vi "add_channel.vi"(8 "error in (no error)":errorcluster, 11 "Channel definition in":T1={"physical Channel"="", "max_input_value"=0.0, "min_input_value"=0.0, "ground_reference"=10083, "translation_factor"=0.0, "translation_offset"=0.0} {"ground_reference" items=["default"=-1, "RSE"=10083, "NRSE"=10078, "Differential"=10106, "Pseudodifferential"=12529]}) -> (0 "error out":errorcluster, 2 "Canceled":bool, 3 "Channel definition out":T1={"physical Channel"="", "max_input_value"=0.0, "min_input_value"=0.0, "ground_reference"=10083, "translation_factor"=0.0, "translation_offset"=0.0} {"ground_reference" items=["default"=-1, "RSE"=10083, "NRSE"=10078, "Differential"=10106, "Pseudodifferential"=12529]})   [LabVIEW 2012, in "SignalReaderCN091129DAQmx.lvclass"]
doc: "Collects the information to add/edit an Analog input DAQ channel"
uses:
  SignalReaderCN091129DAQmx.lvclass
  C:/Program Files (x86)/National Instruments/LabVIEW 2010/resource/objmgr/daqmx.rc
  TypeDefs/channel_definition_cluster.ctl
panel:
  in  "ground reference":i32(ring)=10083 items=["default"=-1, "RSE"=10083, "NRSE"=10078, "Differential"=10106, "Pseudodifferential"=12529]
  in  "Add":bool
  in  "cancel":bool
  in  "voltage range":i32(ring) items=["-0.20 - 0.20", "-1.00 - 1.00", "-5.00 - 5.00", "-10.00 - 10.00"]
  in  "translation offset":dbl
  in  "translation factor":dbl
  in  "Physical Channel":tag
  # "Add / Edit analog input channel"
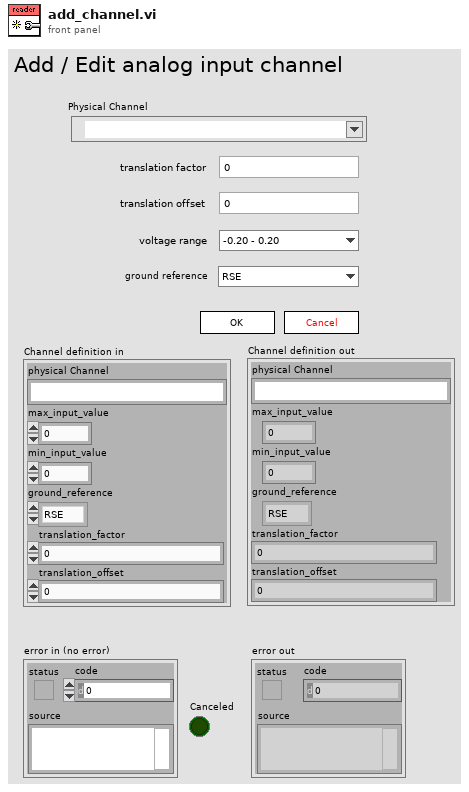
[diagram p1: front panel]
types:
  T1 = typedef "SignalReaderCN091129DAQmx.lvclass/channel_definition_cluster.ctl" = cluster{"physical Channel":string, "max_input_value":dbl, "min_input_value":dbl, "ground_reference":i32, "translation_factor":dbl, "translation_offset":dbl}
  T2 = cluster{"AI.Voltage.Rngs[0]":dbl, "AI.Voltage.Rngs[1]":dbl}
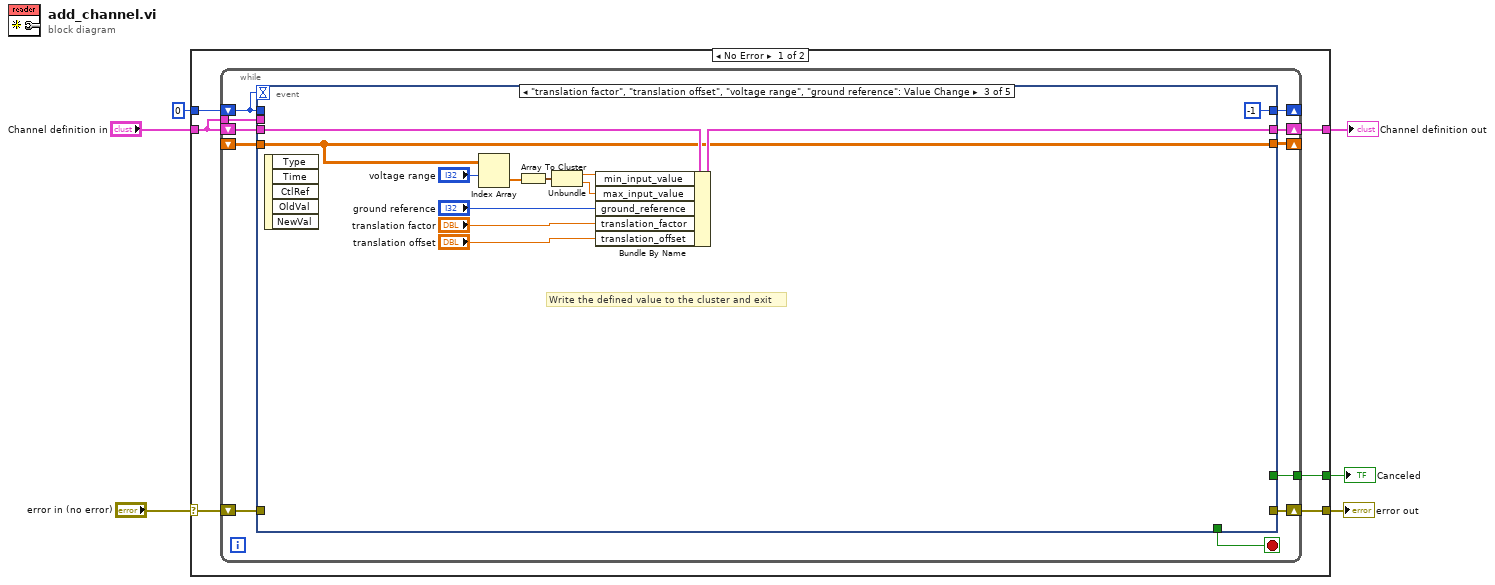
[diagram p0: block diagram]
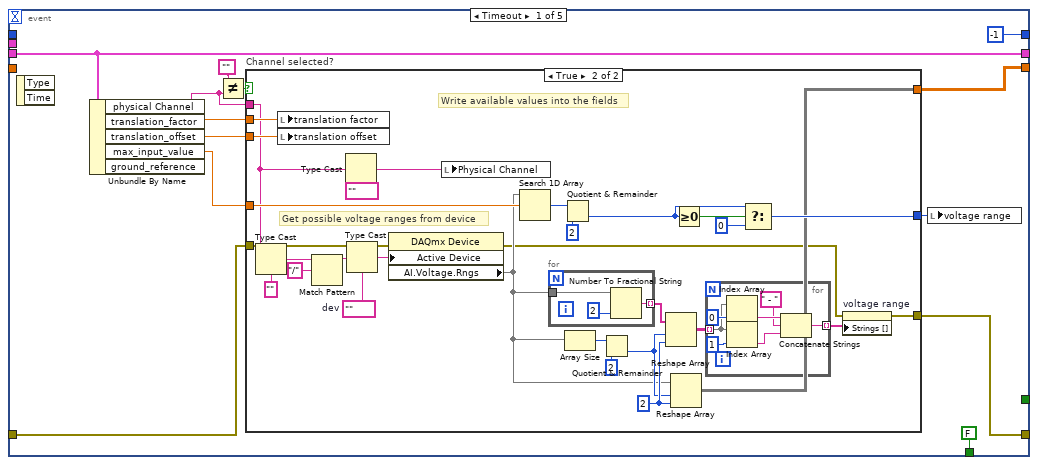
[diagram p2: hidden frame]
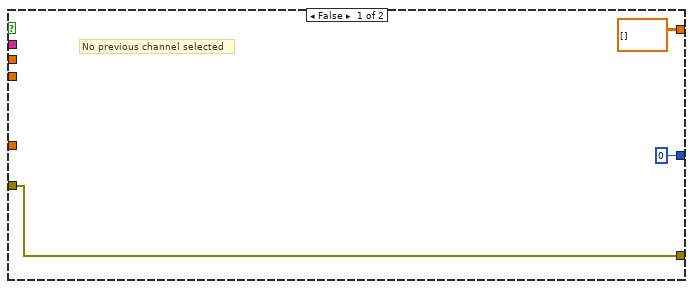
[diagram p3: hidden frame]
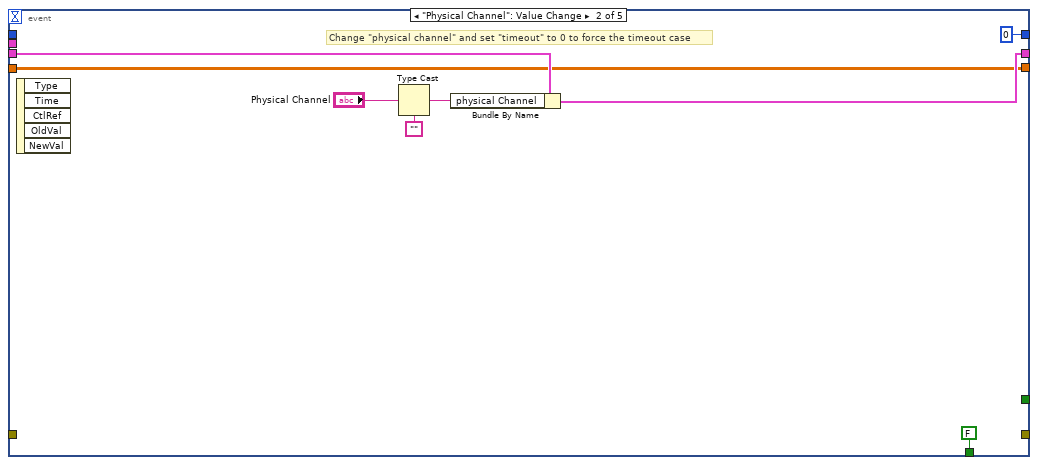
[diagram p4: hidden frame]
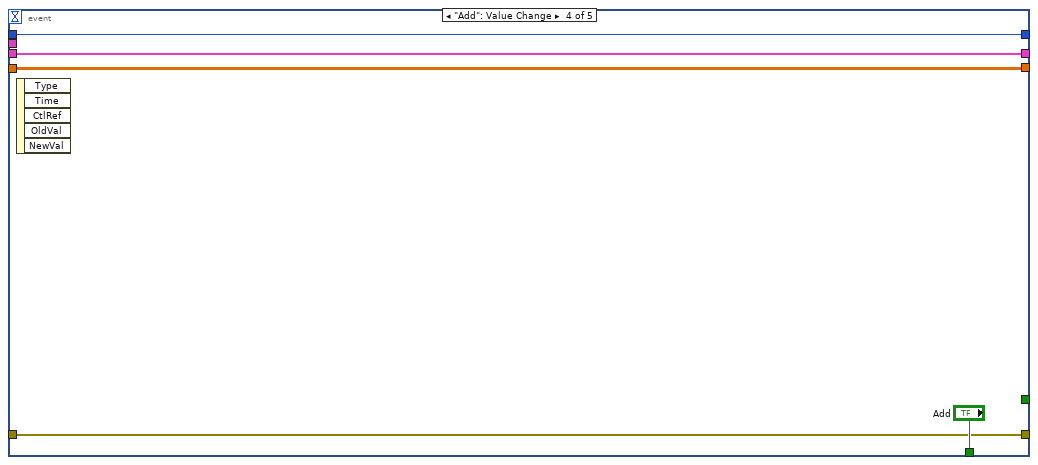
[diagram p5: hidden frame]
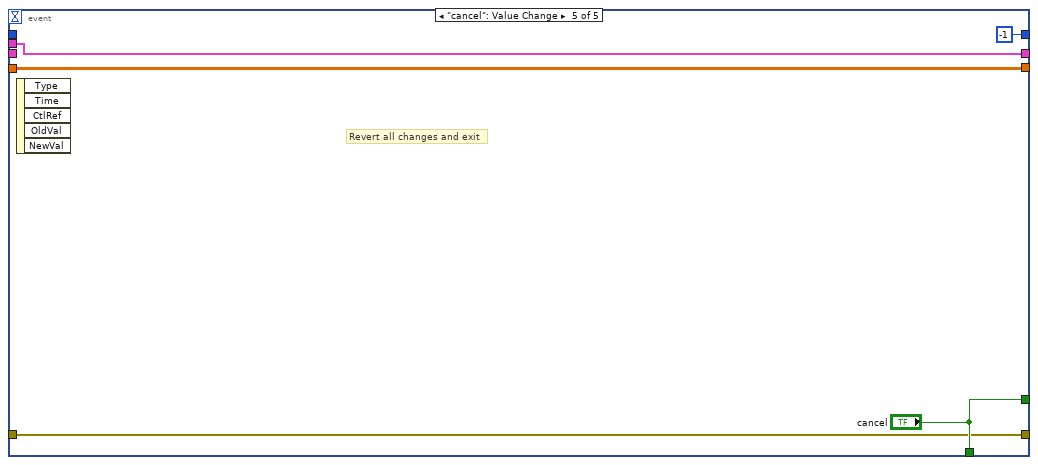
[diagram p6: hidden frame]
diagram:
  n1 = case shown="No Error" "error in (no error)" {
    selector: "error in (no error)" -> [w11 w111]
    tunnel: [w10 w111] -> w5
    tunnel: "Channel definition in" -> [w8 w110]
    tunnel: [w9 w110] -> w3
    tunnel: 0 -> [w12 _]
    tunnel: [w7 _] -> w1
    frame No Error {
      n2 = while {
        shift-right: [w18] -> w10
        shift-left: w11 -> [w19]
        shift-right: [w22] -> _
        shift-left: w12 -> [w23]
        shift-right: [w20] -> w9
        shift-left: w8 -> [w21]
        shift-right: [w17] -> _
        shift-left: _ -> [w16]
        tunnel: w8 -> [w14]
        tunnel: [w13] -> w7
        stop <- w15 stop-if-true
        n3 = event shown="[2] \"translation factor\", \"translation offset\", \"voltage range\", \"ground reference\": Value Change" {
          selector: _ -> [_ _ _ _ _]
          dyn-events: _ -> [_ _ _ _ _]
          timeout: w23 -> [_ _ _ _ _]
          tunnel: [-1 0 -1 w101 -1] -> w22
          tunnel: w23 -> [_ _ _ w101 _]
          tunnel: w21 -> [w35 w87 w99 w102 _]
          tunnel: [w35 w86 w90 w102 w107] -> w20
          tunnel: w19 -> [w30 _ _ w100 w105]
          tunnel: [w26 _ _ w100 w105] -> w18
          tunnel: [w27 w85 w89 w103 w109] -> w17
          tunnel: w16 -> [_ w85 w89 w103 w109]
          tunnel: [FALSE ("Add") FALSE ("Add") _ "Add" "cancel"] -> w15
          tunnel: w14 -> [_ _ _ _ w107]
          tunnel: [_ _ _ _ "cancel"] -> w13
          event Timeout {
            n4 = event-data() -> ()  [unwired: 1 in, 2 out]
            n5 = Unbundle By Name(w35) -> ("physical Channel"=w33:string, "translation_factor"=w32:dbl, "translation_offset"=w31:dbl, "max_input_value"=w29:dbl)  [unwired: 1 out]
            n6 = Not Equal?(x="", y=w33) -> (x != y?=w34:bool)
            n7 = case "Channel selected?" shown="True" w34 {
              tunnel: w33 -> [_ w42]
              tunnel: w32 -> [_ w69]
              tunnel: w31 -> [_ w68]
              tunnel: w30 -> [w37 w61]
              tunnel: w29 -> [_ w58]
              tunnel: [0 w51] -> w28
              tunnel: [dbl[][] [] ("AI.Voltage.Rngs") w45] -> w27
              tunnel: [w37 w43] -> w26
              frame False {
                # "No previous channel selected"
              }
              frame True {
                w48 = 2 ("dimension size")
                w63 = tag ""  # dev
                # "Get possible voltage ranges from device"
                # "Write available values into the fields"
                n8 = Type Cast(type="", x=w42) -> (*(type *) &x=w66:string)
                n9 = local write "translation factor"(w69) -> ()
                n10 = local write "translation offset"(w68) -> ()
                n11 = Match Pattern(string=w66, regular expression="/") -> (before substring=w64:string)  [unwired: 1 in, 3 out]
                n12 = Type Cast(type=tag "" ("Physical Channel"), x=w42) -> (*(type *) &x=w40:tag)
                n13 = Type Cast(type=w63, x=w64) -> (*(type *) &x=w62:tag)
                n14 = property class="DAQmx Device"(error in=w61, "Active Device"=w62) -> (error out=w44:errorcluster, "AI.Voltage.Rngs"=w46)  [unwired: 1 in, 1 out]
                n15 = local write "Physical Channel"(w40) -> ()
                n16 = Search 1D Array(1D array=w46, element=w58) -> (index of element=w57:i32)  [unwired: 1 in]
                n17 = for {
                  tunnel: w46 -> [w79]
                  tunnel: [w78] -> w55 mode=indexing
                  n18 = Number To Fractional String(number=w79, precision (6)=i16 2) -> (F-format string=w78:string)  [unwired: 2 in]
                }
                n19 = Quotient & Remainder(x=w57, y=2) -> (floor(x/y)=w50:i32)  [unwired: 1 out]
                n20 = Array Size(array=w46) -> (size(s)=w60:i32)
                n21 = Quotient & Remainder(x=w60, y=2) -> (floor(x/y)=w47:i32)  [unwired: 1 out]
                n22 = Reshape Array(w55, w47, w48) -> (w54:string[][])
                n23 = Reshape Array(w46, w47, w48) -> (w45:void[][])
                n24 = Greater Or Equal To 0?(x=w50) -> (x >= 0?=w52:bool)
                n25 = for {
                  tunnel: w54 -> [w73] mode=indexing
                  tunnel: [w70] -> w53 mode=indexing
                  n26 = Index Array(array=w73, index=0) -> (element=w74:string)
                  n27 = Index Array(array=w73, index=1) -> (element=w72:string)
                  n28 = Concatenate Strings(w74, " - " ("string"), w72) -> (w70:string)
                }
                n29 = Select(t=w50, s=w52, f=0) -> (s? t:f=w51:i32)
                n30 = property on="voltage range" class="Ring (strict)"(error in=w44, "Strings []"=w53) -> (error out=w43:errorcluster)  [unwired: 1 in, 1 out]
              }
            }
            n31 = local write "voltage range"(w28) -> ()
          }
          event "Physical Channel": Value Change {
            # "Change \"physical channel\" and set \"timeout\" to 0 to force the timeout case"
            n32 = event-data() -> ()  [unwired: 1 in, 5 out]
            n33 = Type Cast(type="", x="Physical Channel") -> (*(type *) &x=w81:string)
            n34 = Bundle By Name(cluster=w87, "physical Channel"=w81) -> (w86:T1)
          }
          event "translation factor", "translation offset", "voltage range", "ground reference": Value Change {
            # "Write the defined value to the cluster and exit"
            n35 = event-data() -> ()  [unwired: 1 in, 5 out]
            n36 = Index Array(array=w89, index (row)="voltage range") -> (element=w97:dbl[])  [unwired: 1 in]
            n37 = Array To Cluster(array=w97) -> (cluster=w96:T2)
            n38 = Unbundle(w96) -> ("AI.Voltage.Rngs[0]"=w95:dbl, "AI.Voltage.Rngs[1]"=w94:dbl)
            n39 = Bundle By Name(cluster=w99, "min_input_value"=w95, "max_input_value"=w94, "ground_reference"="ground reference", "translation_factor"="translation factor", "translation_offset"="translation offset") -> (w90:T1)
          }
          event "Add": Value Change {
            n40 = event-data() -> ()  [unwired: 1 in, 5 out]
          }
          event "cancel": Value Change {
            # "Revert all changes and exit"
            n41 = event-data() -> ()  [unwired: 1 in, 5 out]
          }
        }
      }
    }
    frame Error {
    }
  }
  "error out" <- w5
  "Channel definition out" <- w3
  "Canceled" <- w1
